vi "is queue invalid.vi"(11 "queues":T1) -> (3 "queue invalid?":bool)   [LabVIEW 2015, in "Queue connection.lvclass"]
uses:
  Queue connection.lvclass
  queue pair.ctl
  message/communicator message.lvclass
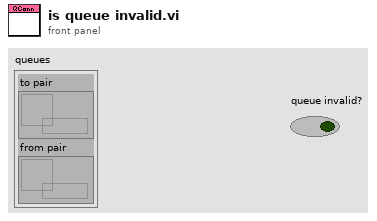
[diagram p1: front panel]
types:
  T1 = typedef "Queue connection.lvclass/queue pair.ctl" = cluster{"to pair":refnum<queue>, "from pair":refnum<queue>}
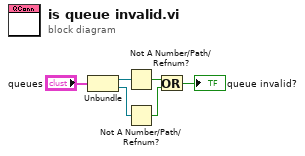
[diagram p0: block diagram]
diagram:
  n1 = Unbundle("queues") -> ("to pair"=w5:refnum<queue>, "from pair"=w6:refnum<queue>)
  n2 = Not A Number/Path/Refnum?(number/path/refnum=w5) -> (NaN/Path/Refnum?=w2:bool)
  n3 = Not A Number/Path/Refnum?(number/path/refnum=w6) -> (NaN/Path/Refnum?=w3:bool)
  n4 = Or(x=w2, y=w3) -> (x .or. y?=→"queue invalid?":bool)
